vi "CreateAndFixVelocity.vi"(10 "Timestep":dbl=0.1, 11 "Points In":dbl[][](array[numeric])) -> (3 "Fixed Vel":dbl[][](array[numeric]))   [LabVIEW 2016]
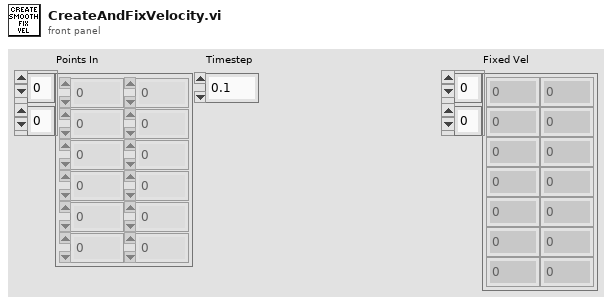
[diagram p1: front panel]
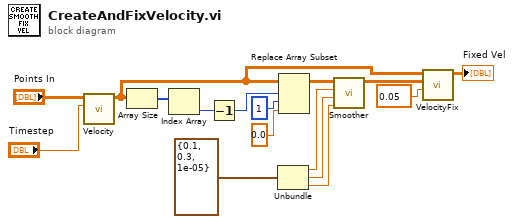
[diagram p0: block diagram]
diagram:
  n1 = call "Velocity.vi"("Timestep"="Timestep", "Points In"="Points In") -> ("Velocity Out"=w13:dbl[][])  [unwired: 9 in]
  n2 = Array Size(array=w13) -> (size(s)=w14:i32[])
  n3 = Index Array(array=w14) -> (element=w15:i32)  [unwired: 1 in]
  n4 = Decrement(x=w15) -> (x-1=w16:i32)
  n5 = Unbundle(cluster{"A":dbl, "B":dbl, "tolerance":dbl} {"A"=0.1, "B"=0.3, "tolerance"=1e-05} ("Smooth Config")) -> ("A"=w5:dbl, "B"=w4:dbl, "tolerance"=w2:dbl)
  n6 = Replace Array Subset(array=w13, new element=0.0 ("new element/subarray"), index (row)=w16, index (col)=1 ("disabled index (col)")) -> (w7:dbl[][])
  n7 = call "Smoother.vi"("tolerance"=w2, "B"=w4, "A"=w5, "Array In"=w7) -> ("Smooth Array"=w6:dbl[][])  [unwired: 7 in]
  n8 = call "VelocityFix.vi"("Tolerance"=0.05, "Smooth Vel"=w6, "Orig Vel"=w13) -> ("Fixed Vel"=→"Fixed Vel":dbl[][])  [unwired: 8 in]
